vi "DAQNavi Read (Counter Frequency 1Chan 1Samp).vi"(8 "error in (no error)":errorcluster, 10 "timeout":dbl=10.0, 11 "task in":i32) -> (0 "error out":errorcluster, 2 "data":dbl, 3 "task out":i32)   [LabVIEW 2020]
uses:
  DAQNavi_LV.dll
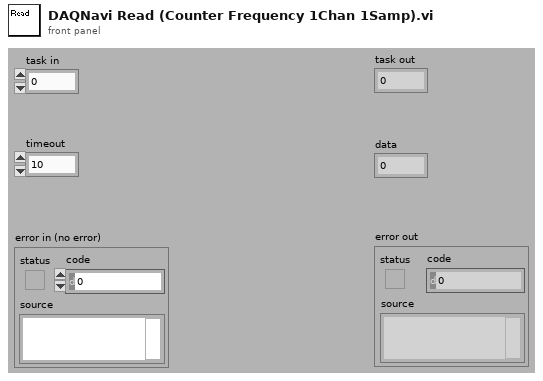
[diagram p1: front panel]
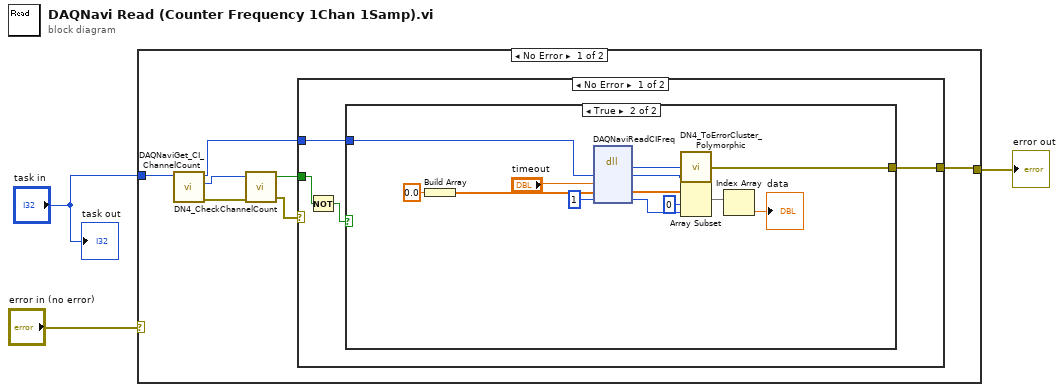
[diagram p0: block diagram]
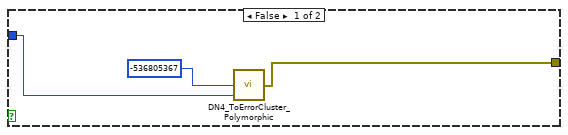
[diagram p2: hidden frame]
diagram:
  n1 = case shown="No Error" "error in (no error)" {
    selector: "error in (no error)" -> [_ w32]
    tunnel: "task in" -> [w9 _]
    tunnel: [w10 w32] -> w1
    frame No Error {
      n2 = call "DAQNaviGet_CI_ChannelCount.vi"("task in"=w9) -> ("error out"=w7:errorcluster, "channel count"=w8:i32, "task out"=w4:i32)  [unwired: 1 in, 7 out]
      n3 = call "DN4_CheckChannelCount.vi"("error out"=w7, "channel count"=w8) -> ("error IO"=w6:errorcluster, "greater than 1?"=w5:bool)  [unwired: 2 out]
      n4 = case shown="No Error" w6 {
        selector: w6 -> [_ w31]
        tunnel: [w14 w31] -> w10
        tunnel: w5 -> [w12 _]
        tunnel: w4 -> [w11 _]
        frame No Error {
          n5 = Not(x=w12) -> (.not. x?=w13:bool)
          n6 = case shown="True" w13 {
            tunnel: [w15 w30] -> w14
            tunnel: w11 -> [w17 w18]
            frame False {
              n7 = call "DN4_ToErrorCluster_Polymorphic.vi"("task id"=w17, "error code"=-536805367) -> ("error out"=w15:errorcluster)  [unwired: 3 out]
            }
            frame True {
              n8 = Build Array(0.0 ("element")) -> (w25:dbl[])
              n9 = dll-call lib="DAQNavi_LV.dll" fn="DAQNaviReadCIFreq"("taskID"=w18, "timeout"="timeout", "freq"=w25, "samples"=u32 1) -> ("return type"=w28:i32, "taskID"=w19:i32, "freq"=w24:dbl[], "samples"=w22:u32)  [unwired: 4 in, 2 out]
              n10 = call "DN4_ToErrorCluster_Polymorphic.vi"("task id"=w19, "error code"=w28) -> ("error out"=w30:errorcluster)  [unwired: 3 out]
              n11 = Array Subset(array=w24, index=0, length=w22) -> (w21:dbl[])
              n12 = Index Array(array=w21) -> (element=→"data":dbl)  [unwired: 1 in]
            }
          }
        }
        frame Error {
        }
      }
    }
    frame Error {
    }
  }
  "error out" <- w1
  "task out" <- "task in"
